vi "ResetConnection.vi"(6 "AuthRegisterClientRequest":T1, 8 "error in (no error)":errorcluster, 11 "service":refnum<class "IcmMessageService.lvclass">) -> (0 "error out":errorcluster, 2 "Header":T2)   [LabVIEW 2016]
uses:
  <vilib>/addons/InsightCM/MessageBus/MessageService/IcmMessageService.lvclass
  <vilib>/addons/InsightCM/MessageBus/Base/controls/KeyValuePair.ctl
  <vilib>/addons/InsightCM/MessageBus/Base/controls/MessageHeader.ctl
  <vilib>/addons/InsightCM/MessageBus/MessageLibrary/Authentication/controls/AuthRegisterClientRequestBody.ctl
panel:
  out "data string":string
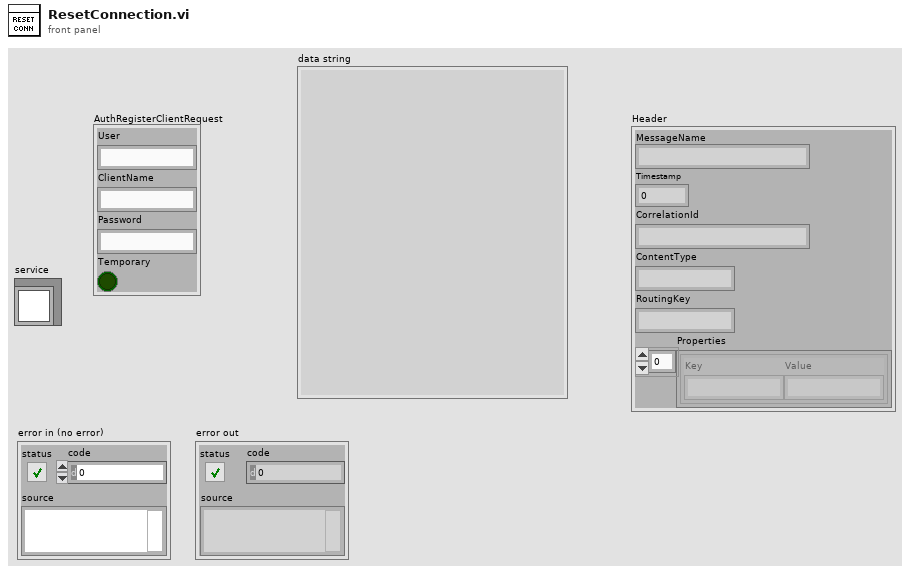
[diagram p1: front panel]
types:
  T1 = typedef "AuthRegisterClientRequestBody.ctl" = cluster{"User":string, "ClientName":string, "Password":string, "Temporary":bool}
  T2 = typedef "MessageHeader.ctl" = cluster{"MessageName":string, "Timestamp":i64, "CorrelationId":string, "ContentType":string, "RoutingKey":string, "Properties":T3[]}
  T3 = typedef "KeyValuePair.ctl" = cluster{"Key":string, "Value":string}
  T4 = typedef "Message.ctl" = cluster{"Header":T2, "Body":u8[]}
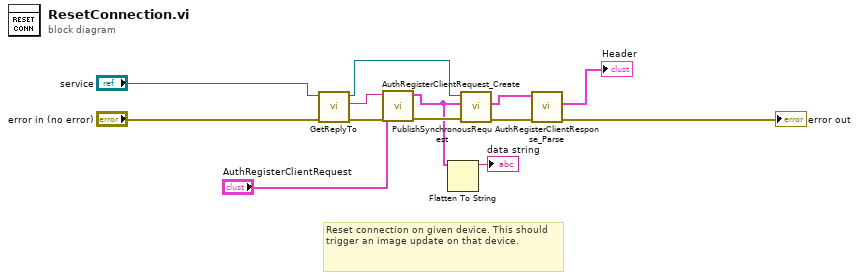
[diagram p0: block diagram]
diagram:
  # "Reset connection on given device. This should trigger an image update on that device."
  n1 = call <vilib>:"GetReplyTo.vi"("error in (no error)"="error in (no error)", "service in"="service") -> ("error out"=w10:errorcluster, "reply to"=w9:string, "service out"=w11:refnum<class "IcmMessageService.lvclass">)  [unwired: 7 in]
  n2 = call <vilib>:"AuthRegisterClientRequest_Create.vi"("error in (no error)"=w10, "AuthRegisterClientRequest"="AuthRegisterClientRequest", "ReplyTo"=w9) -> ("error out"=w6:errorcluster, "Message"=w4:T4)  [unwired: 7 in]
  n3 = Flatten To String(anything=w4) -> (data string=→"data string":string)  [unwired: 3 in, 2 out]
  n4 = call <vilib>:"PublishSynchronousRequest.vi"("error in (no error)"=w6, "request"=w4, "service in"=w11) -> ("error out"=w2:errorcluster, "response"=w8:T4)  [unwired: 6 in, 1 out]
  n5 = call <vilib>:"AuthRegisterClientResponse_Parse.vi"("error in (no error)"=w2, "Message"=w8) -> ("error out"=→"error out":errorcluster, "Header"=→"Header":T2)  [unwired: 7 in, 1 out]
